vi "OriginalClassLine.vi"() -> ()   [LabVIEW 2012]
uses:
  DataBank/DataBank.lvclass
  DataBank/DataBank.lvclass/DataBank.ctl
panel:
  out "DataInStep3InLine2":T1
  out "DataInStep3":T1
  out "DataInStep2":T1
  out "DataInStep1":T1
  # "請見方塊圖說明"
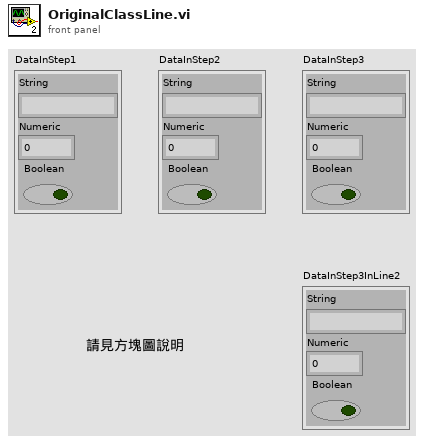
[diagram p1: front panel]
types:
  T1 = cluster{"String":string, "Numeric":i32, "Boolean":bool}
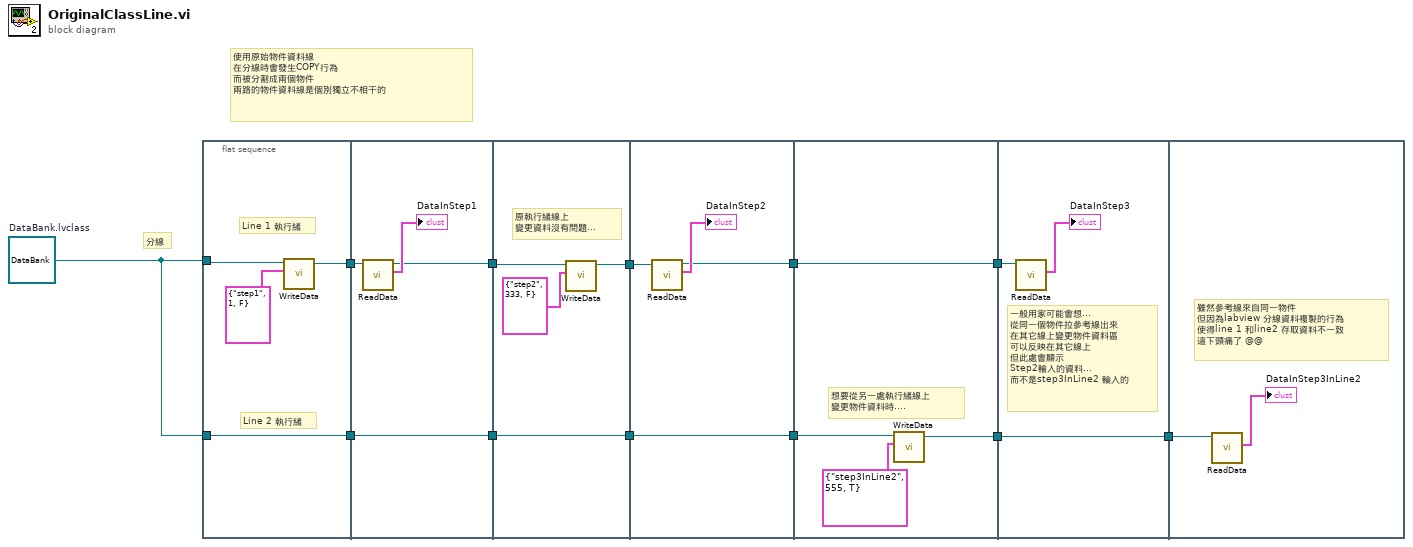
[diagram p0: block diagram]
diagram:
  w7 = refnum<class "DataBank.lvclass"> refnum  # DataBank.lvclass
  # "使用原始物件資料線\n在分線時會發生COPY行為\n而被分割成兩個物件\n兩路的物件資料線是個別獨立不相干的"
  # "分線"
  n1 = flat-sequence {
    tunnel: w7 -> [w16]
    tunnel: [w14] -> w12
    tunnel: [w13] -> w8
    tunnel: w7 -> [w13]
    tunnel: w12 -> [w20]
    tunnel: [w18] -> w11
    tunnel: [w17] -> w10
    tunnel: w8 -> [w17]
    tunnel: w11 -> [w23]
    tunnel: w10 -> [w21]
    tunnel: [w22] -> w9
    tunnel: [w21] -> w5
    tunnel: w9 -> [w27]
    tunnel: [w26] -> w6
    tunnel: w5 -> [w26]
    tunnel: [w25] -> w4
    tunnel: w6 -> [w31]
    tunnel: w4 -> [w30]
    tunnel: [w30] -> w3
    tunnel: [w29] -> w2
    tunnel: w3 -> [w34]
    tunnel: w2 -> [w33]
    tunnel: [w33] -> w1
    tunnel: w1 -> [w36]
    frame #0 {
      # "Line 2 執行緒"
      # "Line 1 執行緒"
      n2 = call "WriteData.vi"("Data"=T1 {"String"="step1", "Numeric"=1, "Boolean"=FALSE}, "DataBank in"=w16) -> ("DataBank out"=w14:refnum<class "DataBank.lvclass">)  [unwired: 8 in, 1 out]
    }
    frame #1 {
      n3 = call "ReadData.vi"("DataBank in"=w20) -> ("Data"=→"DataInStep1":T1, "DataBank out"=w18:refnum<class "DataBank.lvclass">)  [unwired: 8 in, 1 out]
    }
    frame #2 {
      # "原執行緒線上\n變更資料沒有問題..."
      n4 = call "WriteData.vi"("Data"=T1 {"String"="step2", "Numeric"=333, "Boolean"=FALSE}, "DataBank in"=w23) -> ("DataBank out"=w22:refnum<class "DataBank.lvclass">)  [unwired: 8 in, 1 out]
    }
    frame #3 {
      n5 = call "ReadData.vi"("DataBank in"=w27) -> ("Data"=→"DataInStep2":T1, "DataBank out"=w25:refnum<class "DataBank.lvclass">)  [unwired: 8 in, 1 out]
    }
    frame #4 {
      # "想要從另一處執行緒線上\n變更物件資料時...."
      n6 = call "WriteData.vi"("Data"=T1 {"String"="step3InLine2", "Numeric"=555, "Boolean"=TRUE}, "DataBank in"=w31) -> ("DataBank out"=w29:refnum<class "DataBank.lvclass">)  [unwired: 8 in, 1 out]
    }
    frame #5 {
      # "一般用家可能會想...\n從同一個物件拉參考線出來\n在其它線上變更物件資料區\n可以反映在其它線上\n但此處會顯示\nStep2輸入的資料...\n而不是step3InLine2 輪入的"
      n7 = call "ReadData.vi"("DataBank in"=w34) -> ("Data"=→"DataInStep3":T1)  [unwired: 8 in, 2 out]
    }
    frame #6 {
      # "雖然參考線來自同一物件\n但因為labview 分線資料複製的行為\n使得line 1 和line2 存取資料不一致\n這下頭痛了 @@"
      n8 = call "ReadData.vi"("DataBank in"=w36) -> ("Data"=→"DataInStep3InLine2":T1)  [unwired: 8 in, 2 out]
    }
  }
